vi "libssh2_sftp_fsync.vi"(8 "error in (no error)":errorcluster, 11 "sftp handle":T1) -> (0 "error out":errorcluster)   [LabVIEW 2013, in "libssh2.lvlib"]
doc: "Flush a file handle to disk."
uses:
  libssh2.lvlib
  SFTP Handle Refnum.ctl
  Acquire SFTP.vi
  Release SFTP.vi
  Acquire Session.vi
  Release Session.vi
  Not An SFTP Handle Refnum.vi
  <vilib>/Utility/error.llb/Error Cluster From Error Code.vi
  Global Settings.vi
  Read SFTP Handle Refnum.vi
  Read SFTP Refnum.vi
  Read Session Refnum.vi
  <vilib>/Utility/semaphor.llb/Acquire Semaphore.vi
  <vilib>/Utility/semaphor.llb/Release Semaphore.vi
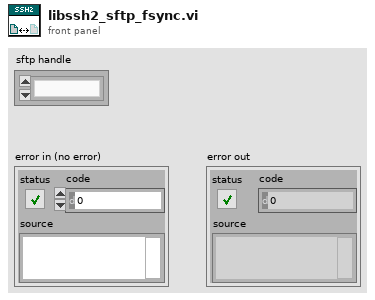
[diagram p1: front panel]
types:
  T1 = typedef "libssh2.lvlib/SFTP Handle Refnum.ctl" = refnum<k1>
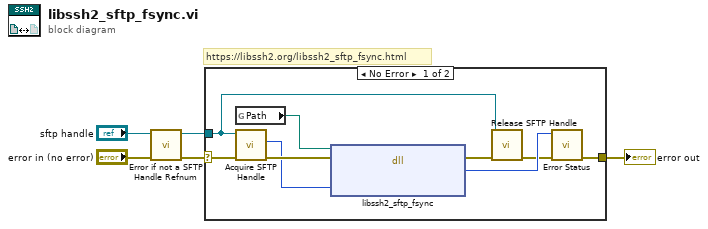
[diagram p0: block diagram]
diagram:
  # "https://libssh2.org/libssh2_sftp_fsync.html"
  n1 = call "Error if not a SFTP Handle Refnum.vi"("error in (no error)"="error in (no error)", "sftp handle"="sftp handle") -> ("error out"=w4:errorcluster, "sftp handle out"=w3:T1)  [unwired: 8 in]
  n2 = case shown="No Error" w4 {
    selector: w4 -> [w13 w15]
    tunnel: w3 -> [w6 _]
    tunnel: [w9 w15] -> w2
    frame No Error {
      n3 = global read "Global Settings.vi" "Path"() -> (w14:path)
      n4 = call "Acquire SFTP Handle.vi"("error in (no error)"=w13, "sftp handle"=w6) -> ("error out"=w12:errorcluster, "LIBSSH2_SFTP_HANDLE*"=w11:u64)  [unwired: 8 in]
      n5 = dll-call lib="?" fn="libssh2_sftp_fsync"(path in=w14, error in=w12, "handle"=w11) -> (error out=w10:errorcluster, "return value"=w8:i32)  [unwired: 2 in, 1 out]
      n6 = call "Release SFTP Handle.vi"("error in (no error)"=w10, "sftp handle"=w6) -> ("error out"=w7:errorcluster)  [unwired: 9 in]
      n7 = call "Error Status.vi"("error in (no error)"=w7, "return value"=w8) -> ("error out"=w9:errorcluster)  [unwired: 8 in, 1 out]
    }
    frame Error {
    }
  }
  "error out" <- w2
